vi "DiffDrivePoseEst_Kalman_F_Callback.vi"(9 "U":T1, 10 "X":T1, 11 "ExtraPassedData":variant) -> (0 "Error":bool, 3 "Result":T1)   [LabVIEW 2019, in "Trajectory_Library.lvlib"]
doc: "Internal function used by DiffDrivePoseEst_Update routines to pass to the Kalman filter Predict routine.\n\nInputs:\n - ExtraPassedData -- Variant of extra data used by this function. (This value is not used.)\n - X -- X matrix\n - U -- U matrix\n\nOutputs:\n - Result -- Resulting matrix\n - Error -- If TRUE, an error occured."
uses:
  Trajectory_Library.lvlib
  <vilib>/Analysis/Matrix/Datatypes/RealMatrix.ctl
  <vilib>/Analysis/baseanly.llb/Real A x B.vi
  MatBuilder_Create.vi
  <vilib>/Analysis/NI_AALBase.lvlib
  <vilib>/Analysis/Matrix/NI_Matrix.lvlib
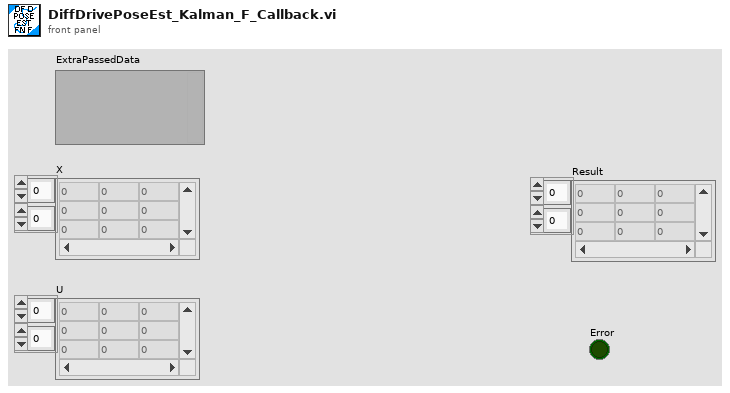
[diagram p1: front panel]
types:
  T1 = typedef "NI_Matrix.lvlib/RealMatrix.ctl" = dbl[][]
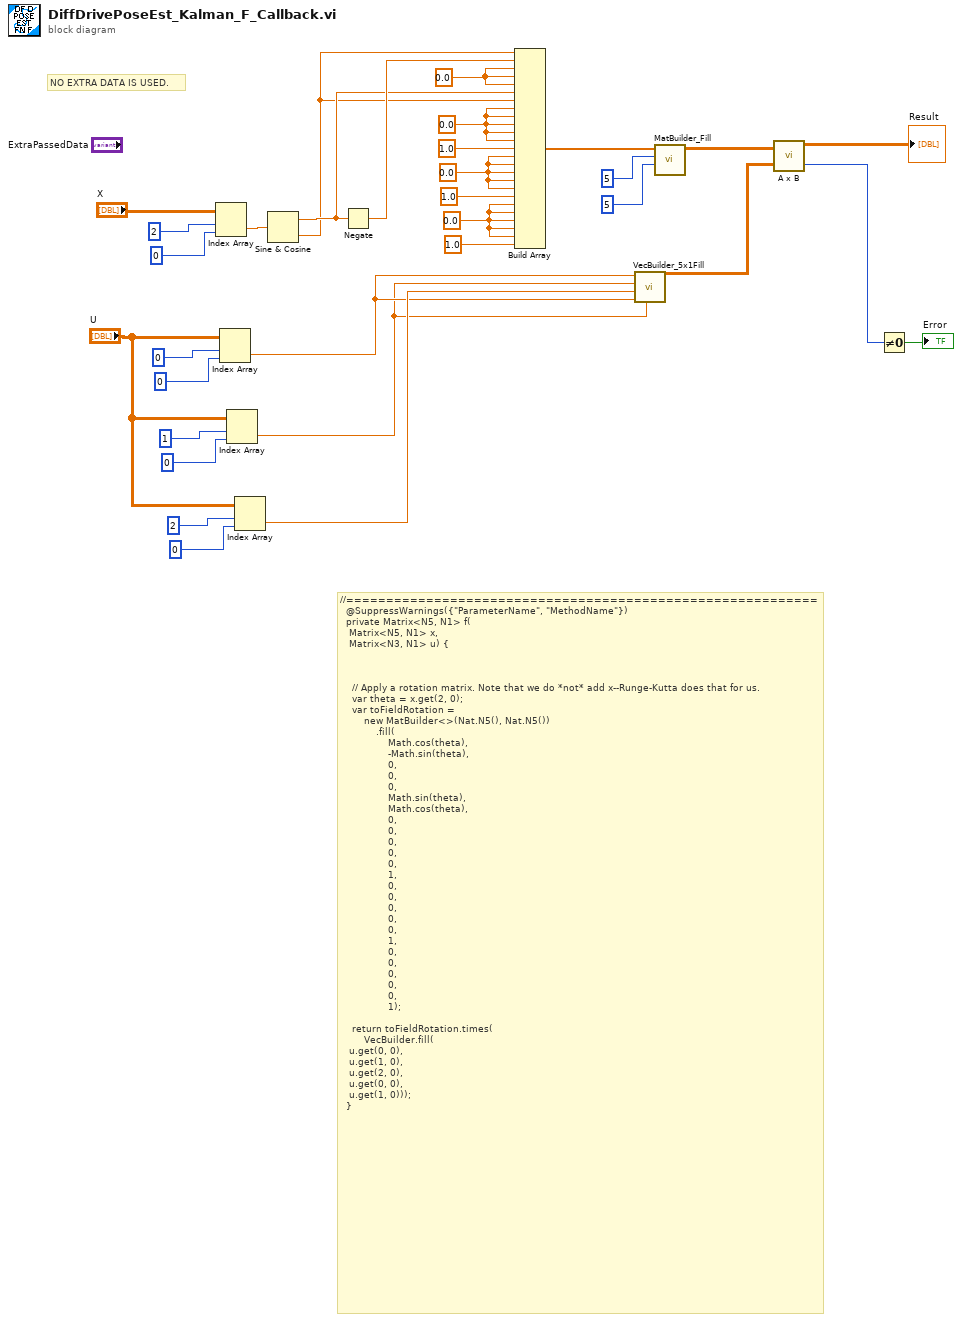
[diagram p0: block diagram]
diagram:
  w13 = 0.0 ("element")
  w15 = 0.0 ("element")
  w17 = 0.0 ("element")
  w20 = 0.0 ("element")
  # "NO EXTRA DATA IS USED."
  # "//===========================================================\n  @SuppressWarnings({\"ParameterName\", \"MethodName\"})\n  private Matrix<N5, N1> f(\n\t\t\tMatrix<N5, N1> x, \n\t\t\tMatrix<N3, N1> u) {\n\n\n\n    // Apply a rotation matrix. Note that we do *not* add x--Runge-Kutta does that for us.\n    var theta = x.get(2, 0);\n    var toFieldRotation =\n        new MatBuilder<>(Nat.N5(), Nat.N5())\n            .fill(\n                Math.cos(theta),\n                -Math.sin(theta),\n                0,\n                0,\n                0,\n                Math.sin(theta),\n                Math.cos(theta),\n                0,\n                0,\n                0,\n                0,\n                0,\n                1,\n                0,\n                0,\n                0,\n                0,\n                0,\n                1,\n                0,\n                0,\n                0,\n                0,\n                0,\n                1);\n\n    return toFieldRotation.times(\n        VecBuilder.fill(  \n\t\t\tu.get(0, 0), \n\t\t\tu.get(1, 0), \n\t\t\tu.get(2, 0), \n\t\t\tu.get(0, 0), \n\t\t\tu.get(1, 0)));\n  }"
  n1 = Index Array(array="X", index (row)=2, index (col)=0) -> (element=w22:dbl)
  n2 = Index Array(array="U", index (row)=0, index (col)=0) -> (element=w2:dbl)
  n3 = Index Array(array="U", index (row)=1, index (col)=0) -> (element=w1:dbl)
  n4 = Index Array(array="U", index (row)=2, index (col)=0) -> (element=w3:dbl)
  n5 = Sine & Cosine(0:w22) -> (1:w19:dbl, 2:w18:dbl)
  n6 = Negate(x=w19) -> (-x=w21:dbl)
  n7 = Build Array(w18, w21, w20, w20, w20, w19, w18, w17, w17, w17, w17, w17, 1.0 ("element"), w15, w15, w15, w15, w15, 1.0 ("element"), w13, w13, w13, w13, w13, 1.0 ("element")) -> (w11:dbl[])
  n8 = call "VecBuilder_5x1Fill.vi"("R4"=w1, "R3"=w2, "R2"=w3, "R1"=w1, "R0"=w2) -> ("output matrix"=w29:T1)  [unwired: 6 in]
  n9 = call "MatBuilder_Fill.vi"("Columns"=5, "Rows"=5, "Value List"=w11) -> ("output matrix"=w30:T1)  [unwired: 8 in]
  n10 = call-poly <vilib>:"A x B.vi"("B"=w29, "A"=w30) -> ("error"=w27:i32, "A x B"=→"Result":T1)
  n11 = Not Equal To 0?(x=w27) -> (x != 0?=→"Error":bool)
